vi "YokoGS200 Set Output.vi"(8 "error in (no error)":errorcluster, 9 "Output State":bool, 11 "VISA Rsrc":refnum<visa-resource-name>="SR530") -> (0 "error out":errorcluster, 3 "VISA Rsrc Out":refnum<visa-resource-name>="GPIB0::12::INSTR")   [LabVIEW 2012]
uses:
  <userlib>/Yoko GS200/YokoGS200 lvl_states ctl.ctl
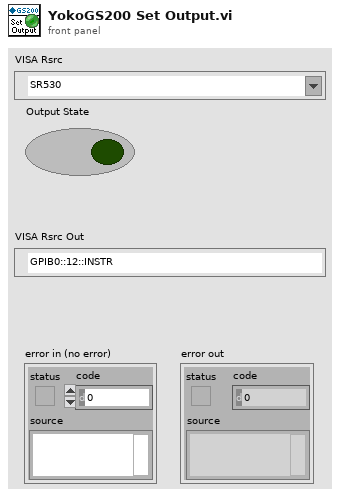
[diagram p1: front panel]
types:
  T1 = typedef "YokoGS200 lvl_states ctl.ctl" = enum16{"Send Command", "Check Errors", "End"}
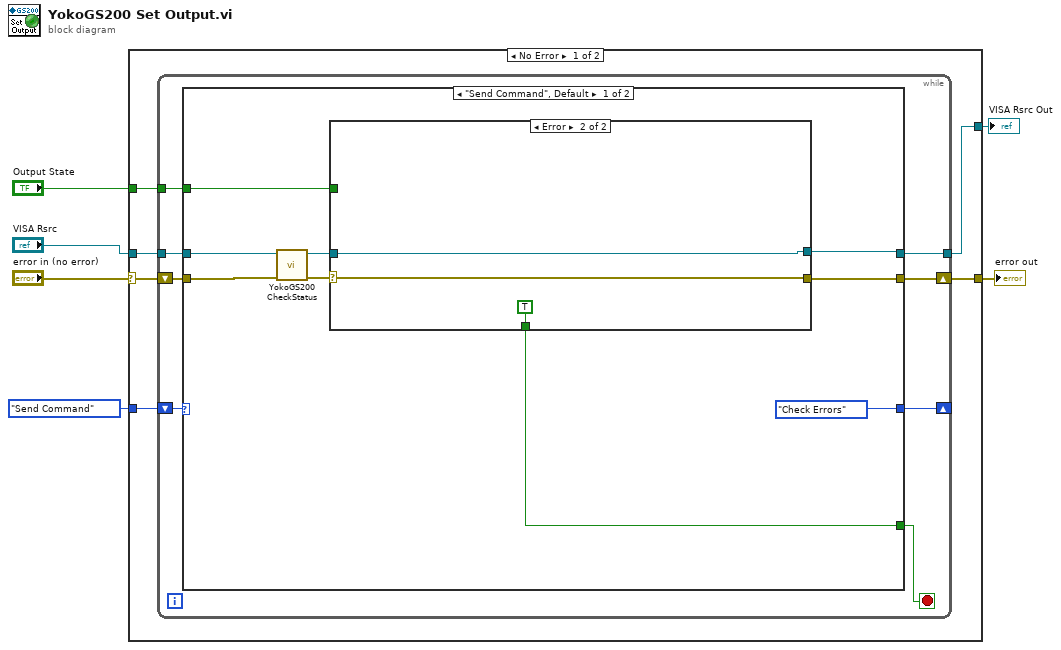
[diagram p0: block diagram]
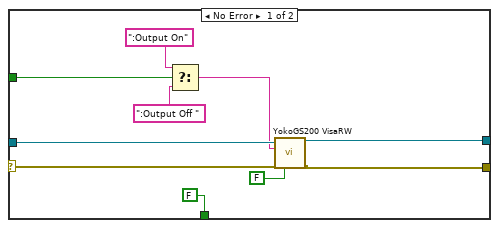
[diagram p2: hidden frame]
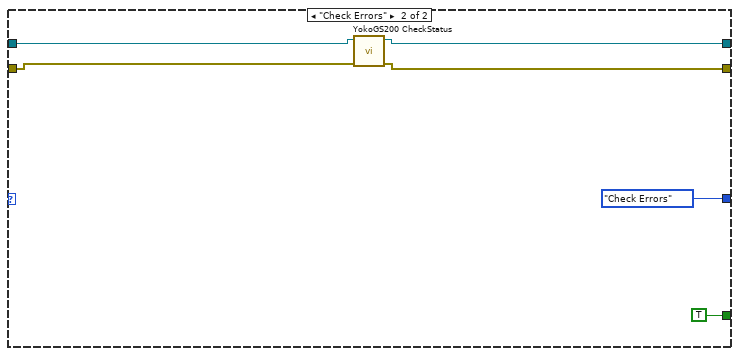
[diagram p3: hidden frame]
diagram:
  n1 = case shown="No Error" "error in (no error)" {
    selector: "error in (no error)" -> [w12 w49]
    tunnel: "VISA Rsrc" -> [w11 w50]
    tunnel: [w7 w49] -> w4
    tunnel: [w10 w50] -> w3
    tunnel: "Output State" -> [w9 _]
    tunnel: YokoGS200_lvl_states_ctl."Send Command" ("Level State") -> [w8 _]
    frame No Error {
      n2 = while {
        tunnel: w11 -> [w19]
        tunnel: [w18] -> w10
        tunnel: w9 -> [w17]
        shift-right: [w15] -> _
        shift-left: w8 -> [w16]
        shift-right: [w13] -> w7
        shift-left: w12 -> [w20]
        stop <- w14 stop-if-true
        n3 = case shown="\"Send Command\", Default" w16 {
          tunnel: w20 -> [w27 w48]
          tunnel: w19 -> [w28 w47]
          tunnel: [w24 w46] -> w18
          tunnel: [w23 w45] -> w13
          tunnel: w17 -> [w29 _]
          tunnel: [YokoGS200_lvl_states_ctl."Check Errors" ("Level State") YokoGS200_lvl_states_ctl."Check Errors" ("Level State")] -> w15
          tunnel: [w21 TRUE] -> w14
          frame "Send Command", Default {
            n4 = call <userlib>:"YokoGS200 CheckStatus.vi"("error in (no error)"=w27, "VISA Rsrc"=w28) -> ("error out"=w26:errorcluster, "VISA Rsrc Out"=w25:refnum<visa-resource-name>)  [unwired: 6 in, 2 out]
            n5 = case shown="Error" w26 {
              selector: w26 -> [w36 w42]
              tunnel: w29 -> [w39 _]
              tunnel: w25 -> [w34 w41]
              tunnel: [w32 w41] -> w24
              tunnel: [w31 w42] -> w23
              tunnel: [FALSE TRUE] -> w21
              frame No Error {
                n6 = Select(t=":Output On" ("initial string"), s=w39, f=":Output Off " ("initial string")) -> (s? t:f=w33:string)
                n7 = call <userlib>:"YokoGS200 VisaRW.vi"("VISA Rsrc"=w34, "ChaineCom"=w33, "error in (no error)"=w36, "Lecture?(T)"=FALSE) -> ("VISA Rsrc Out"=w32:refnum<visa-resource-name>, "error out"=w31:errorcluster)  [unwired: 7 in, 3 out]
              }
              frame Error {
              }
            }
          }
          frame "Check Errors" {
            n8 = call <userlib>:"YokoGS200 CheckStatus.vi"("error in (no error)"=w48, "VISA Rsrc"=w47) -> ("error out"=w45:errorcluster, "VISA Rsrc Out"=w46:refnum<visa-resource-name>)  [unwired: 6 in, 2 out]
          }
        }
      }
    }
    frame Error {
    }
  }
  "error out" <- w4
  "VISA Rsrc Out" <- w3
